vi "Magnet Check On.vi"() -> (1 "magarray":T1(array[cluster]), 2 "ready?":bool)   [LabVIEW 2009, in "Magnet.lvclass"]
uses:
  Magnet.lvclass
  Global/Mag Array.vi
  Global/Magnet Names.vi
  Global/Power Supply.vi
  Global/Temp Controller.vi
  Global/Level Meter.vi
panel:
  out "time":u32
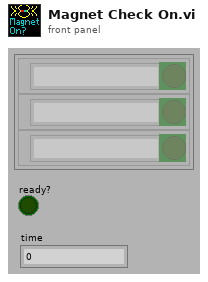
[diagram p1: front panel]
types:
  T1 = cluster{"name":string, "on?":bool, "abbrev":string}[]
  T2 = cluster{"dispname":string, bool, "abbrev":string}[]
  T3 = typedef "PSIO.ctl" = cluster{"Address":T4, "Version":enum16{"PS", "IPS"}}
  T4 = typedef "OxfordAddress.ctl" = cluster{"Com Port":i32, "ISOBUS Address":i32, "GPIB Address":i16, "Communication":enum16{"RS232", "ISOBUS", "GPIB", "Gateway"}}
  T5 = typedef "ITCIO.ctl" = cluster{"Address":T4, "Version":T6, "Ch 1 dec places":i16, "Ch 2 dec places":i16, "Ch 3 dec places":i16, "Ch1 Name":string, "Ch2 Name":string, "Ch3 Name":string}
  T6 = typedef "ITCVersion.ctl" = enum16{"ITC502", "ITC503", "ITC601"}
  T7 = cluster{"Address":T4, "ILM Name":string, "Display Channel":i32[]}
  T8 = cluster{"dispname":string, "selection":bool, "abbrev":string}
  T9 = cluster{"dispname":string, "selection":bool, "abbrev":string}[]
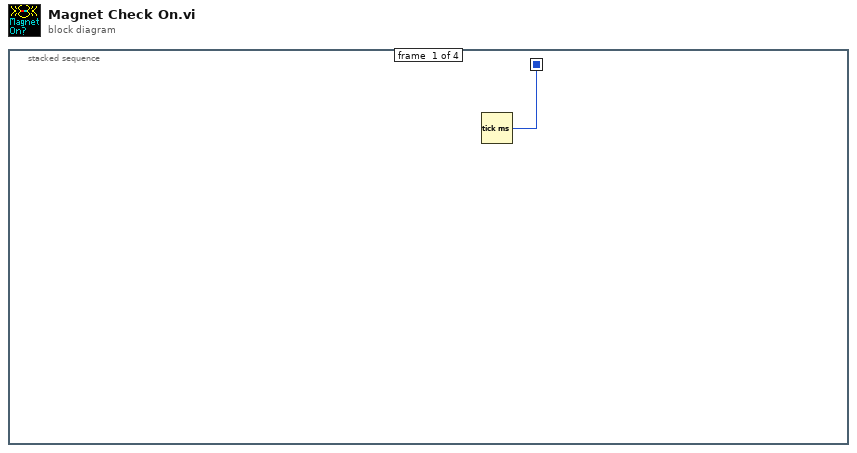
[diagram p0: block diagram]
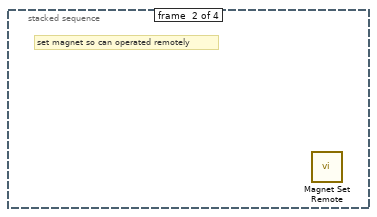
[diagram p2: hidden frame]
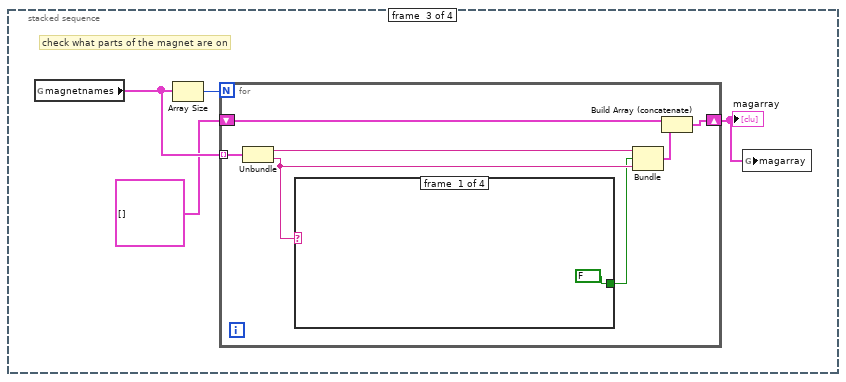
[diagram p3: hidden frame]
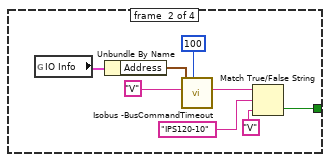
[diagram p4: hidden frame]
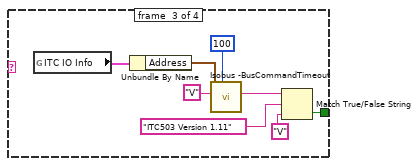
[diagram p5: hidden frame]
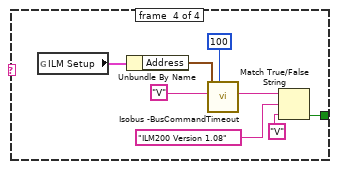
[diagram p6: hidden frame]
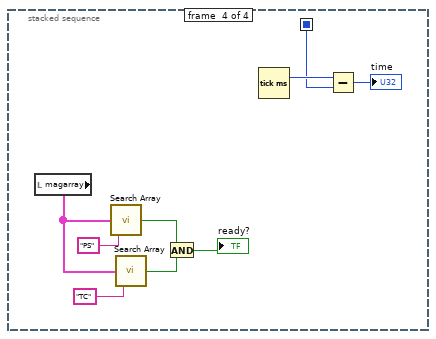
[diagram p7: hidden frame]
diagram:
  n1 = stacked-sequence {
    seq-local: [w1 _ _ _] -> [_ _ _ w45]
    frame #0 {
      n2 = Tick Count (ms)() -> (millisecond timer value=w1:u32)
    }
    frame #1 {
      # "set magnet so can operated remotely"
      n3 = call "Magnet Set Remote.vi"() -> ()  [unwired: 1 out]
    }
    frame #2 {
      # "check what parts of the magnet are on"
      n4 = global read "Magnet Names.vi" "magnetnames"() -> (w4:cluster{"dispname":string, "abbrev":string}[])
      n5 = Array Size(array=w4) -> (size(s)=w5:i32)
      n6 = for {
        N: w5 -> [_]
        tunnel: w4 -> [w12] mode=indexing
        shift-right: [w8] -> w2
        shift-left: T2 [] -> [w10]
        n7 = Unbundle(w12) -> ("dispname"=w11:string, "abbrev"=w7:string)
        n8 = case shown="\"TC\"" w7 {
          tunnel: [FALSE w14 w22 w30] -> w6
          frame #0 {
          }
          frame #1 {
            n9 = global read "Power Supply.vi" "IO Info"() -> (w15:T3)
            n10 = Unbundle By Name(w15) -> ("Address"=w19:T4)
            n11 = call "Isobus -BusCommandTimeout.vi"("Timeout (ms)"=100, "Command"="V", "Address"=w19) -> ("Reply"=w21:string)  [unwired: 5 out]
            n12 = Match True/False String(2:"V", 3:"IPS120-10", 4:w21) -> (0:w14:bool)  [unwired: 1 out]
          }
          frame #2 {
            n13 = global read "Temp Controller.vi" "ITC IO Info"() -> (w23:T5)
            n14 = Unbundle By Name(w23) -> ("Address"=w27:T4)
            n15 = call "Isobus -BusCommandTimeout.vi"("Timeout (ms)"=100, "Command"="V", "Address"=w27) -> ("Reply"=w29:string)  [unwired: 5 out]
            n16 = Match True/False String(2:"V", 3:"ITC503 Version 1.11", 4:w29) -> (0:w22:bool)  [unwired: 1 out]
          }
          frame #3 {
            n17 = global read "Level Meter.vi" "ILM Setup"() -> (w31:T7)
            n18 = Unbundle By Name(w31) -> ("Address"=w35:T4)
            n19 = call "Isobus -BusCommandTimeout.vi"("Timeout (ms)"=100, "Command"="V", "Address"=w35) -> ("Reply"=w37:string)  [unwired: 5 out]
            n20 = Match True/False String(2:"V", 3:"ILM200 Version 1.08", 4:w37) -> (0:w30:bool)  [unwired: 1 out]
          }
        }
        n21 = Bundle("dispname"=w11, "selection"=w6, "abbrev"=w7) -> (w9:T8)  [unwired: 1 out]
        n22 = Build Array (concatenate)(w10, w9) -> (w8:T9)
      }
      "magarray" <- w2
      n23 = global write "Mag Array.vi" "magarray"(w2) -> ()
    }
    frame #3 {
      n24 = local read "magarray"() -> (w43:T1)
      n25 = call "Search Array.vi"("abbrev"="PS", "instrarray"=w43) -> ("on?"=w40:bool)  [unwired: 3 out]
      n26 = call "Search Array.vi"("abbrev"="TC", "instrarray"=w43) -> ("on?"=w39:bool)  [unwired: 3 out]
      n27 = And(x=w40, y=w39) -> (x .and. y?=→"ready?":bool)
      n28 = Tick Count (ms)() -> (millisecond timer value=w46:u32)
      n29 = Subtract(x=w46, y=w45) -> (x-y=→"time":u32)
    }
  }
